vi "Add Icons From Pictures.vi"(8 "error in (no error)":errorcluster, 9 "Names":string[](array[string]), 10 "Pictures":picture[](array[picture]), 11 "Toolbar Control in":refnum<class "Toolbar Control.lvclass">) -> (0 "error out":errorcluster, 3 "Toolbar Control out":refnum<class "Toolbar Control.lvclass">)   [LabVIEW 2011, in "Toolbar Control.lvclass"]
doc: "This VI will add the image <B>Pictures</B> to the <B>Toolbar Control in</B> at the available location or if specified by <B>Icon Index (Next)</B>. The name of the icon is specified by <B>Icon Names</B>.\n\n-------------\nDeveloped by Brian Hoover (hooovahh)"
uses:
  Toolbar Control.lvclass
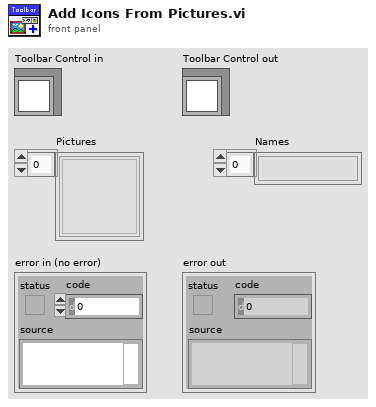
[diagram p1: front panel]
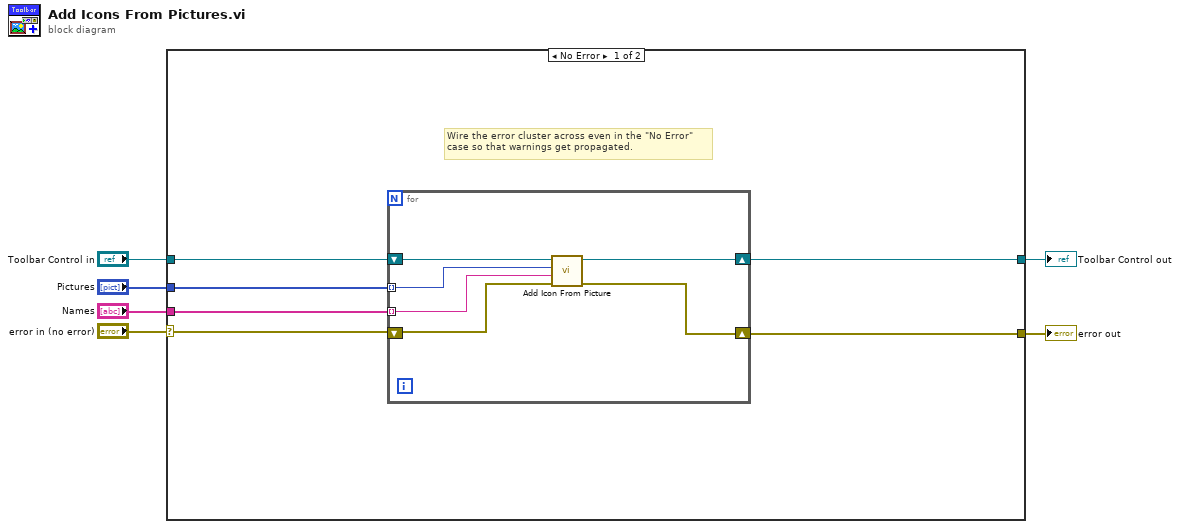
[diagram p0: block diagram]
diagram:
  n1 = case shown="No Error" "error in (no error)" {
    selector: "error in (no error)" -> [w8 w20]
    tunnel: [w7 w20] -> w5
    tunnel: [w11 w19] -> w3
    tunnel: "Toolbar Control in" -> [w12 w19]
    tunnel: "Pictures" -> [w10 _]
    tunnel: "Names" -> [w9 _]
    frame No Error {
      # "Wire the error cluster across even in the \"No Error\"\ncase so that warnings get propagated."
      n2 = for {
        tunnel: w10 -> [w13] mode=indexing
        shift-right: [w17] -> w11
        shift-left: w12 -> [w18]
        tunnel: w9 -> [w16] mode=indexing
        shift-right: [w14] -> w7
        shift-left: w8 -> [w15]
        n3 = call "Add Icon From Picture.vi"("error in (no error)"=w15, "Icon Name"=w16, "Picture"=w13, "Toolbar Control in"=w18) -> ("error out"=w14:errorcluster, "Toolbar Control out"=w17:refnum<class "Toolbar Control.lvclass">)  [unwired: 6 in]
      }
    }
    frame Error {
    }
  }
  "error out" <- w5
  "Toolbar Control out" <- w3
